vi "cha desc constructor.vi"(11 "init_scan_cha_desc":T1) -> (3 "ad_scan_cha_desc":T2)   [LabVIEW 2021, in "libad4.lvlib"]
doc: "Helper function to aid in the construction of an ad_scan_cha_desc cluster/struct."
uses:
  <userlib>/libad4/controls/ad scan cha desc.ctl
  <userlib>/libad4/controls/init scan cha desc.ctl
  <userlib>/libad4/libad4.lvlib
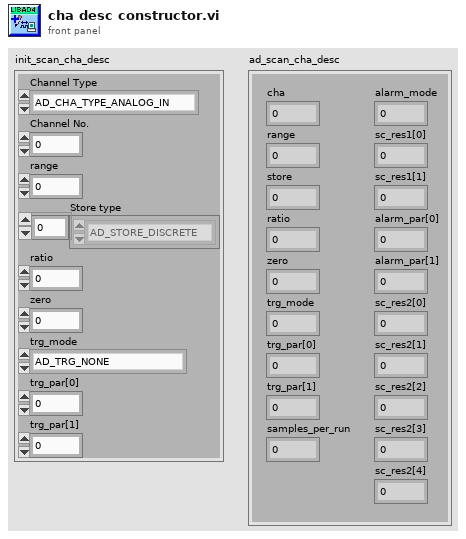
[diagram p1: front panel]
types:
  T1 = typedef "libad4.lvlib/init scan cha desc.ctl" = cluster{"Channel Type":enum16{"AD_CHA_TYPE_ANALOG_IN", "AD_CHA_TYPE_ANALOG_OUT", "AD_CHA_TYPE_DIGITAL_IO"}, "Channel No.":i32, "range":i32, "Store type":enum16{"AD_STORE_DISCRETE", "AD_STORE_AVERAGE", "AD_STORE_MIN", "AD_STORE_MAX", "AD_STORE_RMS"}[], "ratio":i32, "zero":u32, "trg_mode":enum16{"AD_TRG_NONE", "AD_TRG_POSITIVE", "AD_TRG_NEGATIVE", "AD_TRG_INSIDE", "AD_TRG_OUTSIDE", "AD_TRG_NEVER"}, "trg_par[0]":u32, "trg_par[1]":u32}
  T2 = typedef "libad4.lvlib/ad scan cha desc.ctl" = cluster{"cha":i32, "range":i32, "store":i32, "ratio":i32, "zero":u32, "trg_mode":u8, "alarm_mode":u8, "sc_res1[0]":u8, "sc_res1[1]":u8, "trg_par[0]":u32, "trg_par[1]":u32, "samples_per_run":i32, "alarm_par[0]":u32, "alarm_par[1]":u32, "sc_res2[0]":u32, "sc_res2[1]":u32, "sc_res2[2]":u32, "sc_res2[3]":u32, "sc_res2[4]":u32}
  T3 = enum16{"AD_CHA_TYPE_ANALOG_IN", "AD_CHA_TYPE_ANALOG_OUT", "AD_CHA_TYPE_DIGITAL_IO"}
  T4 = enum16{"AD_STORE_DISCRETE", "AD_STORE_AVERAGE", "AD_STORE_MIN", "AD_STORE_MAX", "AD_STORE_RMS"}[]
  T5 = enum16{"AD_TRG_NONE", "AD_TRG_POSITIVE", "AD_TRG_NEGATIVE", "AD_TRG_INSIDE", "AD_TRG_OUTSIDE", "AD_TRG_NEVER"}
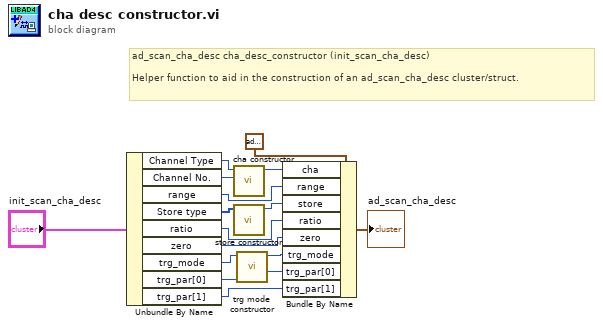
[diagram p0: block diagram]
diagram:
  # "ad_scan_cha_desc cha_desc_constructor (init_scan_cha_desc)\n\nHelper function to aid in the construction of an ad_scan_cha_desc cluster/struct."
  n1 = Unbundle By Name("init_scan_cha_desc") -> ("Channel Type"=w10:T3, "Channel No."=w9:i32, "range"=w8:i32, "Store type"=w7:T4, "ratio"=w6:i32, "zero"=w5:u32, "trg_mode"=w3:T5, "trg_par[0]"=w2:u32, "trg_par[1]"=w1:u32)
  n2 = call <userlib>:"cha constructor.vi"("Channel No."=w9, "Channel Type"=w10) -> ("Channel Number"=w14:i32)  [unwired: 9 in]
  n3 = call <userlib>:"store constructor.vi"("Store type"=w7) -> ("Store ID"=w12:i32)  [unwired: 10 in]
  n4 = call <userlib>:"trg mode constructor.vi"("trg_mode"=w3) -> ("trg_mode out"=w4:u8)  [unwired: 10 in]
  n5 = Bundle By Name(cluster=T2 {"cha"=0, "range"=0, "store"=0, "ratio"=0, "zero"=0, "trg_mode"=0, "alarm_mode"=0, "sc_res1[0]"=0, "sc_res1[1]"=0, "trg_par[0]"=0, "trg_par[1]"=0, "samples_per_run"=0, "alarm_par[0]"=0, "alarm_par[1]"=0, "sc_res2[0]"=0, "sc_res2[1]"=0, "sc_res2[2]"=0, "sc_res2[3]"=0, "sc_res2[4]"=0} ("ad_scan_cha_desc"), "cha"=w14, "range"=w8, "store"=w12, "ratio"=w6, "zero"=w5, "trg_mode"=w4, "trg_par[0]"=w2, "trg_par[1]"=w1) -> (→"ad_scan_cha_desc":T2)
